vi "SENS_CORR_EXT_AUTO_RES.vi"(0 "VISA IN":refnum<visa-resource-name>, 5 "error in":errorcluster, 7 "Channel":i32) -> (14 "VISA Out":refnum<visa-resource-name>, 19 "error out":errorcluster)   [LabVIEW 2018, in "PNA-X.lvlib"]
doc: "SENSe<cnum>:CORRection:EXTension:AUTO:RESet \n1702\n\n(Write-only) Clears old port extension delay and loss data in preparation for acquiring new data. Send \nthis command prior to sending a new series of SENS:CORR:EXT:AUTO:MEAS. If acquiring both \nOPEN and SHORT standards, do not send this command between those acquisitions. \nParameters \n<cnum> Any existing channel number. If unspecified, value is set to 1 \nExamples SENS:CORR:EXT:AUTO:RES \nsense2:correction:extension:auto:reset \nQuery Syntax Not Applicable \nDefault Not Applicable"
uses:
  PNA-X.lvlib
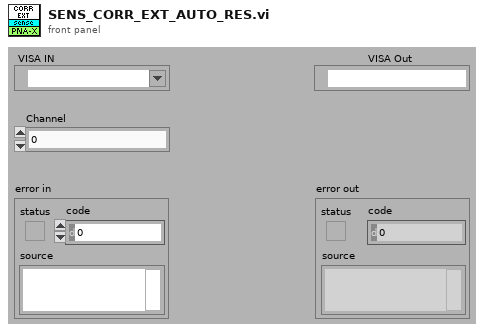
[diagram p1: front panel]
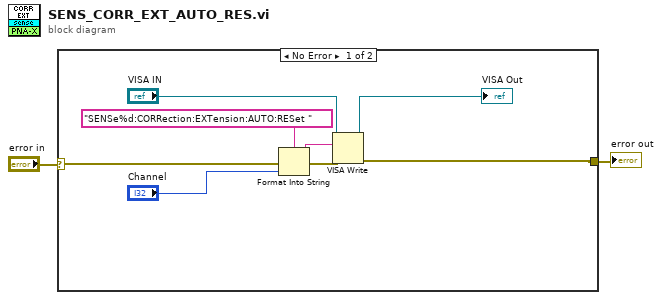
[diagram p0: block diagram]
diagram:
  n1 = case shown="No Error" "error in" {
    selector: "error in" -> [w10 w11]
    tunnel: [w5 w11] -> w1
    frame No Error {
      n2 = Format Into String(format string="SENSe%d:CORRection:EXTension:AUTO:RESet " ("Cmdline"), error in=w10, "Channel") -> (resulting string=w8:string, error out=w9:errorcluster)  [unwired: 1 in]
      n3 = VISA Write(VISA resource name="VISA IN", write buffer=w8, error in (no error)=w9) -> (VISA resource name out=→"VISA Out":refnum<visa-resource-name>, error out=w5:errorcluster)  [unwired: 1 out]
    }
    frame Error {
    }
  }
  "error out" <- w1
